vi "General_Global Stop.vi"(3 "Complete":bool, 4 "Set":T1) -> (1 "Output":T1)   [LabVIEW 2009]
uses:
  Controls/Bool_Otagon Stop Button no latch.ctl
panel:
  out "Parent Vi Name":string
  out "using stop":string[](array[string])
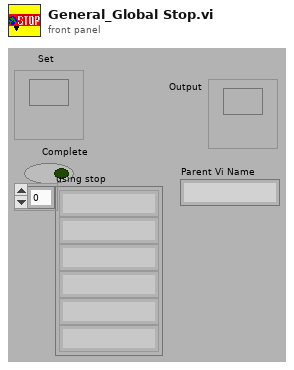
[diagram p1: front panel]
types:
  T1 = typedef "Bool_Otagon Stop Button no latch.ctl" = bool
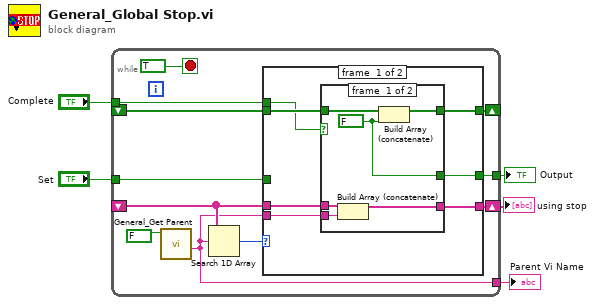
[diagram p0: block diagram]
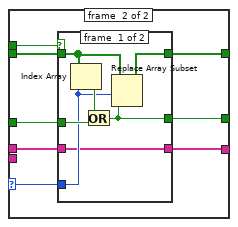
[diagram p3: hidden frame]
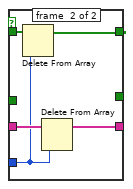
[diagram p4: hidden frame]
diagram:
  n1 = while {
    tunnel: "Complete" -> [w10]
    tunnel: "Set" -> [w16]
    shift-right: [w15] -> _
    shift-left: _ -> [w14]
    shift-right: [w12] -> w2
    shift-left: _ -> [w9]
    tunnel: [w11] -> w3
    tunnel: [w6] -> w1
    stop <- TRUE stop-if-true
    n2 = call "General_Get Parent.vi"("Get Ref? (t)"=FALSE ("Get ref? (t)")) -> ("Parent Vi Name Out"=w6:string)  [unwired: 8 in, 2 out]
    n3 = Search 1D Array(1D array=w9, element=w6) -> (index of element=w13:i32)  [unwired: 1 in]
    n4 = case shown="-1" w13 {
      selector: w13 -> [_ w36]
      tunnel: w16 -> [_ w39]
      tunnel: [w22 w38] -> w15
      tunnel: w14 -> [w23 w37]
      tunnel: w6 -> [w19 _]
      tunnel: w9 -> [w21 w34]
      tunnel: [w20 w33] -> w12
      tunnel: [w18 w32] -> w11
      tunnel: w10 -> [w17 w35]
      frame #0 {
        n5 = case shown="False" w17 {
          tunnel: w23 -> [w29 w31]
          tunnel: [w28 w31] -> w22
          tunnel: w21 -> [w27 w30]
          tunnel: [w26 w30] -> w20
          tunnel: w19 -> [w25 _]
          tunnel: [w24 _] -> w18
          frame #0 {
            w24 = FALSE
            n6 = Build Array (concatenate)(w27, w25) -> (w26:string[])
            n7 = Build Array (concatenate)(w29, w24) -> (w28:bool[])
          }
          frame #1 {
          }
        }
      }
      frame #1 {
        n8 = case shown="False" w35 {
          tunnel: w39 -> [w46 _]
          tunnel: [w45 w50] -> w38
          tunnel: w37 -> [w44 w51]
          tunnel: w36 -> [w42 w47]
          tunnel: [w41 w48] -> w33
          tunnel: w34 -> [w41 w49]
          tunnel: [w40 _] -> w32
          frame #0 {
            n9 = Index Array(array=w44, index=w42) -> (element=w43:bool)
            n10 = Or(x=w43, y=w46) -> (x .or. y?=w40:T1)
            n11 = Replace Array Subset(array=w44, new element=w40, index=w42) -> (w45:bool[])
          }
          frame #1 {
            n12 = Delete From Array(array=w51, index=w47) -> (array with subset deleted=w50:bool[])  [unwired: 1 in, 1 out]
            n13 = Delete From Array(array=w49, index=w47) -> (array with subset deleted=w48:string[])  [unwired: 1 in, 1 out]
          }
        }
      }
    }
  }
  "Output" <- w3
  "using stop" <- w2
  "Parent Vi Name" <- w1
